vi "POST Parameters.vi"(8 "error in (no error)":errorcluster, 9 "parameters":cluster{"name":string, "value":string}[](array[cluster]), 10 "relative URL":string, 11 "eLab in":refnum<class "PL eLabFTW Client.lvclass">) -> (0 "error out":errorcluster, 2 "response body":string, 3 "eLab out":refnum<class "PL eLabFTW Client.lvclass">)   [LabVIEW 2015, in "PL eLabFTW Client.lvclass"]
doc: "Performs POST request with the specified parameters and returns the response body."
uses:
  PL eLabFTW Client.lvclass
  <vilib>/httpClient/MultipartData.ctl
  PL eLabFTW Client.lvclass/PL eLabFTW Client.ctl
  <vilib>/httpClient/LabVIEWHTTPClient.lvlib
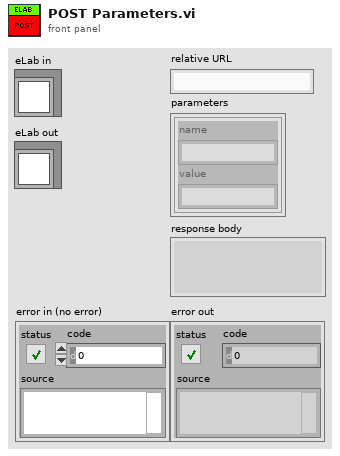
[diagram p1: front panel]
types:
  T1 = typedef "LabVIEWHTTPClient.lvlib/MultipartData.ctl" = cluster{"Name":string, "Value":string, "File":path, "Filename":string, "MIME type":string}
  T2 = typedef "LabVIEWHTTPClient.lvlib/ClientHandle.ctl" = refnum<k1>
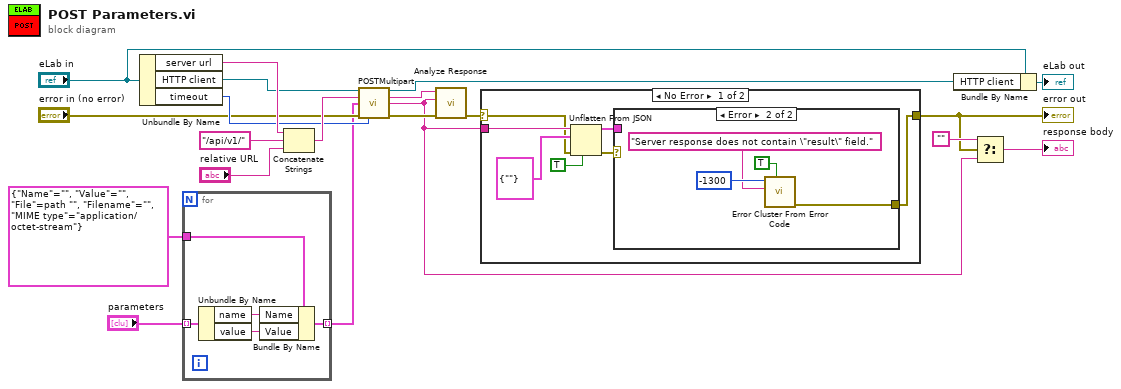
[diagram p0: block diagram]
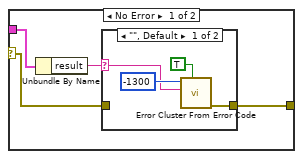
[diagram p2: hidden frame]
diagram:
  n1 = Unbundle By Name("eLab in") -> ("server url"=w20:string, "HTTP client"=w10:T2, "timeout"=w17:i32)
  n2 = for {
    tunnel: T1 {"Name"="", "Value"="", "File"=path "", "Filename"="", "MIME type"="application/octet-stream"} ("Element") -> [w25]
    tunnel: "parameters" -> [w24] mode=indexing
    tunnel: [w21] -> w1 mode=indexing
    n3 = Unbundle By Name(w24) -> ("name"=w23:string, "value"=w22:string)
    n4 = Bundle By Name(cluster=w25, "Name"=w23, "Value"=w22) -> (w21:T1)
  }
  n5 = Concatenate Strings(w20, "/api/v1/" ("string"), "relative URL") -> (w18:string)
  n6 = call <vilib>:"POSTMultipart.vi"("client handle"=w10, "url"=w18, "data"=w1, "error in (no error)"="error in (no error)", "timeout (10000)"=w17) -> ("client handle out"=w7:T2, "headers"=w13:string, "body"=w4:string, "error out"=w14:errorcluster)  [unwired: 7 in]
  n7 = call "Analyze Response.vi"("error in (no error)"=w14, "body"=w4, "headers"=w13) -> ("error out"=w6:errorcluster)  [unwired: 8 in]
  n8 = case shown="No Error" w6 {
    selector: w6 -> [w26 w46]
    tunnel: w4 -> [w32 _]
    tunnel: [w28 w46] -> w5
    frame No Error {
      n9 = Unflatten From JSON(JSON string=w32, type and defaults=cluster{"result":string} {"result"=""}, default null elements? (F)=TRUE, error in (no error)=w26) -> (value=w27:cluster{"result":string}, error out=w29:errorcluster)  [unwired: 3 in]
      n10 = case shown="Error" w29 {
        selector: w29 -> [w34 _]
        tunnel: [w33 w42] -> w28
        tunnel: w27 -> [w36 _]
        frame No Error {
          n11 = Unbundle By Name(w36) -> ("result"=w35:string)
          n12 = case shown="\"\", Default" w35 {
            selector: w35 -> [w38 _]
            tunnel: w34 -> [_ w41]
            tunnel: [w37 w41] -> w33
            frame "", Default {
              n13 = call <vilib>:"Error Cluster From Error Code.vi"("show call chain? (False)"=TRUE, "error message (\"\")"=w38, "error code (0)"=-1300) -> ("error out"=w37:errorcluster)  [unwired: 6 in]
            }
            frame "success" {
            }
          }
        }
        frame Error {
          n14 = call <vilib>:"Error Cluster From Error Code.vi"("show call chain? (False)"=TRUE, "error message (\"\")"="Server response does not contain \"result\" field." ("format string"), "error code (0)"=-1300) -> ("error out"=w42:errorcluster)  [unwired: 6 in]
        }
      }
    }
    frame Error {
    }
  }
  "error out" <- w5
  n15 = Bundle By Name(cluster="eLab in", "HTTP client"=w7) -> (→"eLab out":refnum<class "PL eLabFTW Client.lvclass">)
  n16 = Select(t="", s=w5, f=w4) -> (s? t:f=→"response body":string)
